vi "CRYStep Repeat check.vi"(10 "In String Array":string[](array[string]), 11 "In String for Compare":string) -> (3 "Out String Array":string[](array[string]))   [LabVIEW 2013]
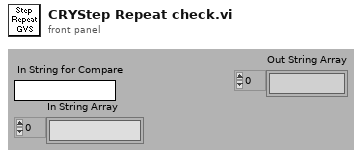
[diagram p1: front panel]
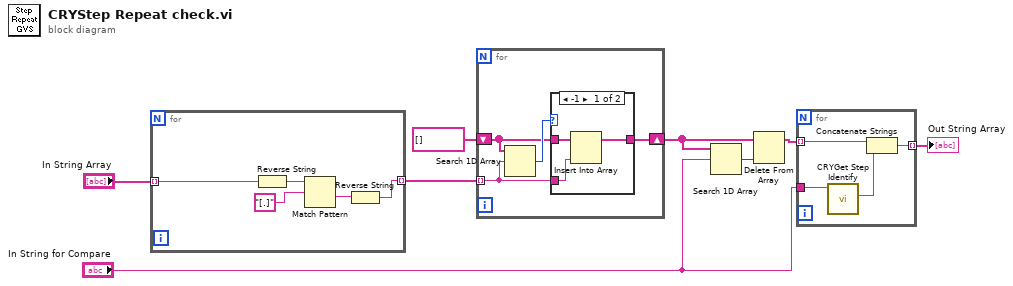
[diagram p0: block diagram]
diagram:
  n1 = for {
    tunnel: "In String Array" -> [w12] mode=indexing
    tunnel: [w9] -> w8 mode=indexing
    n2 = Reverse String(1:w12) -> (0:w11:string)
    n3 = Match Pattern(string=w11, regular expression="[.]") -> (after substring=w10:string)  [unwired: 4 out]
    n4 = Reverse String(1:w10) -> (0:w9:string)
  }
  n5 = for {
    tunnel: w8 -> [w16] mode=indexing
    shift-right: [w15] -> w7
    shift-left: string[] [] ("Out String Array") -> [w14]
    n6 = Search 1D Array(1D array=w14, element=w16) -> (index of element=w17:i32)  [unwired: 1 out]
    n7 = case shown="-1" w17 {
      tunnel: w16 -> [w20 _]
      tunnel: [w18 w21] -> w15
      tunnel: w14 -> [w19 w21]
      frame -1 {
        n8 = Insert Into Array(array=w19, new element=w20) -> (w18:string[])  [unwired: 1 in]
      }
      frame Default {
      }
    }
  }
  n9 = Search 1D Array(1D array=w7, element="In String for Compare") -> (index of element=w2:i32)  [unwired: 1 out]
  n10 = Delete From Array(array=w7, index=w2) -> (array with subset deleted=w4:string[])  [unwired: 1 in, 1 out]
  n11 = for {
    tunnel: w4 -> [w25] mode=indexing
    tunnel: "In String for Compare" -> [w24]
    tunnel: [w22] -> w1 mode=indexing
    n12 = call "CRYGet Step Identify.vi"("Category Name In"=w24) -> ("Identfier(Regular Expression)"=w23:string)  [unwired: 3 in, 7 out]
    n13 = Concatenate Strings(w25, w23) -> (w22:string)
  }
  "Out String Array" <- w1
